vi "WFDC Get Reference Images.vi"(0 "IDS Camera Notifier":string="IDS-Camera-Wide Field Drift Correction-1", 2 "Data Save Path":path=path "C:/Users/George Sirinakis/Documents/Microscope Control/Microscope Modules/Wide Field Drift Correction/WFDC Default Data Storage", 7 "Z Stage Notifier":string="Prior-Stage-Sample Z-Dev1/ao0", 11 "Scan Range":dbl=1.0, 13 "Frame per Step":u32=1, 14 "Scan Positions File Name":string="Scan Positions.xml") -> ()   [LabVIEW 2020]
uses:
  Device Library/Cameras/IDS/IDS Controls/IDS Actions.ctl
  Device Library/Stages/Stages Controls/Stage Actions.ctl
  <vilib>/Utility/miscctls.llb/LVPointTypeDef.ctl
  WFDC Controls/WFDC Reference Image Info.ctl
panel:
  out "Wait Bar":i32(slide) scale=0.0..11.0
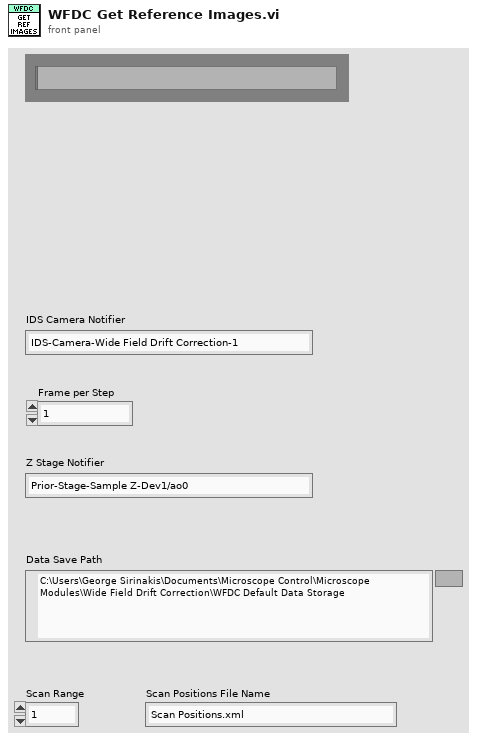
[diagram p1: front panel]
types:
  T1 = typedef "Stage Actions.ctl" = enum16{"Get Position", "MVR", "MOVE", "HALT", "ONTARGET", "ERROR", "REFERENCE", "INIT", "VELOCITY", "STATUS", "EXIT", "HOME", "ZEROPOS", "NANOPOS", "ANALOG", "QUIT"}
  T2 = enum16{"Always On", "Always Off", "Off While Running"}
  T3 = typedef "LVPointTypeDef.ctl" = cluster{"Horizontal":i16, "Vertical":i16}
  T4 = typedef "IDS Actions.ctl" = enum16{"Error Check", "Initialize", "Preview", "Record", "Abort", "Record Settings", "Set Parameter", "Get Parameter", "Set ROI", "Get ROI", "Status", "Quit"}
  T5 = typedef "LVRectTypeDef.ctl" = cluster{"Left":i16, "Top":i16, "Right":i16, "Bottom":i16}
  T6 = typedef "LVBoundsTypeDef.ctl" = cluster{"Width":u32, "Height":u32}
  T7 = typedef "WFDC Reference Image Info.ctl" = cluster{"Image Path":path, "Z Position":dbl, "Number of Frames":u32}
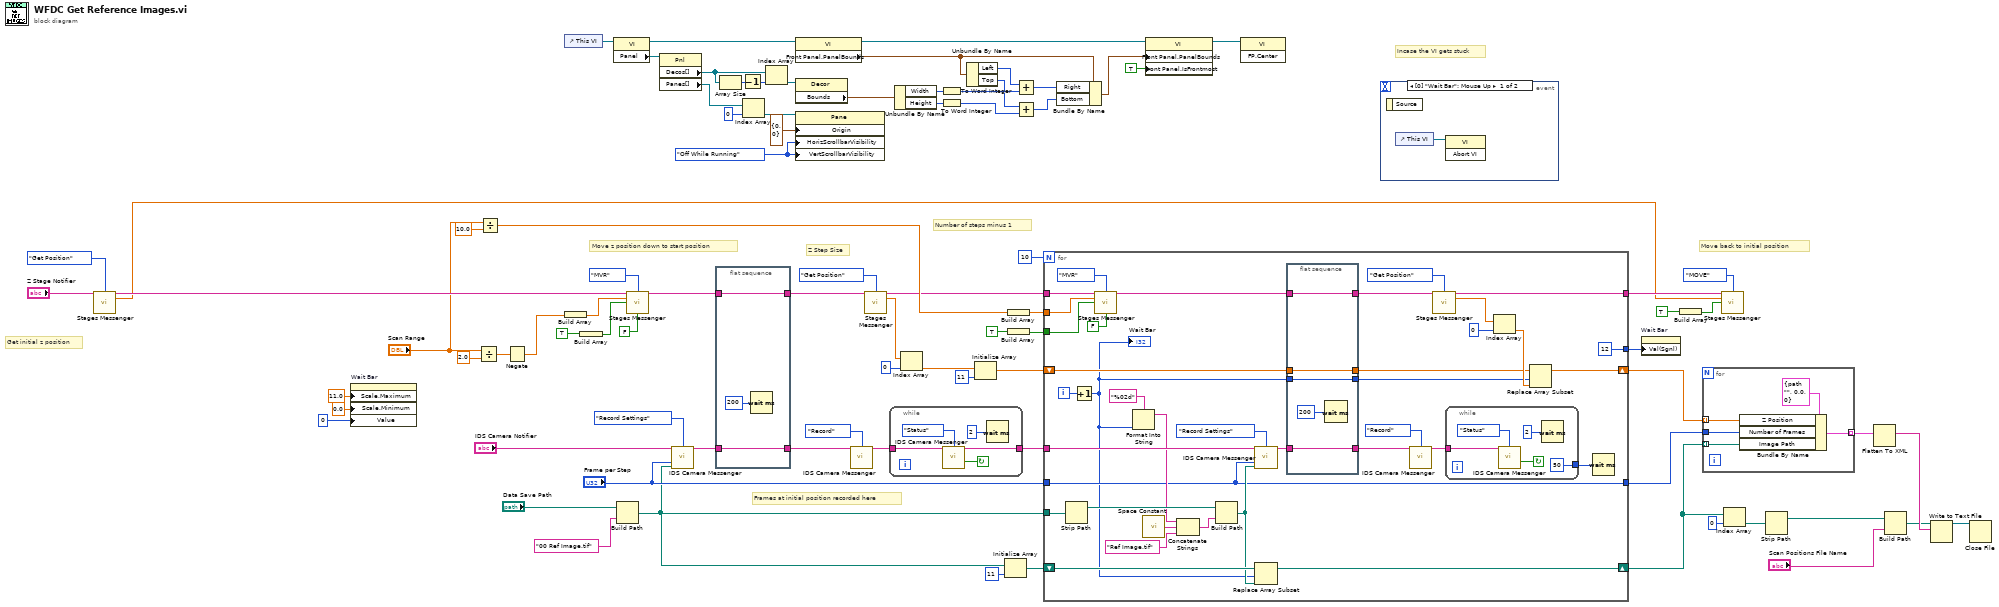
[diagram p0: block diagram]
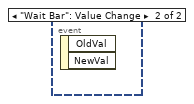
[diagram p2: hidden frame]
diagram:
  w36 = T2."Off While Running" ("Vertical Scrollbar Visibility")
  # "Z Step Size"
  # "Number of steps minus 1"
  # "Frames at initial position recorded here"
  # "Incase the VI gets stuck"
  # "Move back to initial position"
  # "Move z position down to start position"
  # "Get initial z position"
  n1 = call "Stages Messenger.vi"("Stage Notifier Name"="Z Stage Notifier", "Actions"=Stage_Actions."Get Position") -> ("Stage Notifier Name (Dup)"=w77:string, "Positions"=w47:dbl[])  [unwired: 9 in, 3 out]
  n2 = property on="Wait Bar" class="Slide (strict)"("Scale.Maximum"=11.0 ("Scale.Range:Maximum"), "Scale.Minimum"=0.0 ("Scale.Range:Minimum"), "Value"=0 ("Wait Bar")) -> ()  [unwired: 2 in, 2 out]
  n3 = Divide(x="Scan Range", y=2.0) -> (x/y=w13:dbl)
  n4 = Divide(x="Scan Range", y=10.0) -> (x/y=w10:dbl)
  n5 = Negate(x=w13) -> (-x=w14:dbl)
  n6 = control-ref of="This VI"() -> (w19:refnum<vi>)
  n7 = Build Array(w14) -> (w80:dbl[])
  n8 = Build Array(TRUE) -> (w81:bool[])
  n9 = property class="VI"(reference=w19) -> (reference out=w37:refnum<vi>, "Panel"=w30:refnum<vi>)  [unwired: 1 in, 1 out]
  n10 = Build Path(base path="Data Save Path", name or relative path="00 Ref Image.tif") -> (appended path=w59:path)
  n11 = call "Stages Messenger.vi"("Stage Notifier Name"=w77, "Actions"=Stage_Actions."MVR", "Setpoint"=w80, "Axis"=w81, "Exit While Busy?"=FALSE) -> ("Stage Notifier Name (Dup)"=w9:string)  [unwired: 6 in, 4 out]
  n12 = property class="Pnl"(reference=w30) -> ("Decos[]"=w29:refnum<vi>[], "Panes[]"=w33:refnum<vi>[])  [unwired: 1 in, 2 out]
  n13 = call "IDS Camera Messenger.vi"("Notifier Name"="IDS Camera Notifier", "IDS Actions"=IDS_Actions."Record Settings", "# of Frames"="Frame per Step", "File Save Path"=w59) -> ("Notifier Name (Dup)"=w73:string)  [unwired: 6 in, 5 out]
  n14 = flat-sequence {
    tunnel: w9 -> [w89]
    tunnel: [w89] -> w7
    tunnel: w73 -> [w88]
    tunnel: [w88] -> w72
    frame #0 {
      n15 = Wait (ms)(milliseconds to wait=u32 200) -> ()  [unwired: 1 out]
    }
  }
  n16 = Array Size(array=w29) -> (size(s)=w27:i32)
  n17 = Decrement(x=w27) -> (x-1=w28:i32)
  n18 = Index Array(array=w33, index=0) -> (element=w32:refnum<vi>)
  n19 = Index Array(array=w29, index=w28) -> (element=w35:refnum<vi>)
  n20 = property class="VI"(reference=w37) -> (reference out=w39:refnum<vi>, "Front Panel.PanelBounds"=w40:T5)  [unwired: 1 in, 1 out]
  n21 = property class="Decor"(reference=w35) -> ("Bounds"=w38:T6)  [unwired: 1 in, 2 out]
  n22 = property class="Pane"(reference=w32, "Origin"=T3 {"Horizontal"=0, "Vertical"=0}, "HorizScrollbarVisibility"=w36, "VertScrollbarVisibility"=w36) -> ()  [unwired: 1 in, 2 out]
  n23 = call "IDS Camera Messenger.vi"("Notifier Name"=w72, "IDS Actions"=IDS_Actions."Record") -> ("Notifier Name (Dup)"=w49:string)  [unwired: 8 in, 5 out]
  n24 = call "Stages Messenger.vi"("Stage Notifier Name"=w7, "Actions"=Stage_Actions."Get Position") -> ("Stage Notifier Name (Dup)"=w4:string, "Positions"=w6:dbl[])  [unwired: 9 in, 3 out]
  n25 = while {
    tunnel: w49 -> [w93]
    tunnel: [w90] -> w48
    stop <- w92 continue-if-true
    n26 = call "IDS Camera Messenger.vi"("Notifier Name"=w93, "IDS Actions"=IDS_Actions."Status") -> ("Notifier Name (Dup)"=w90:string, "Running?"=w92:bool)  [unwired: 8 in, 4 out]
    n27 = Wait (ms)(milliseconds to wait=u32 2) -> ()  [unwired: 1 out]
  }
  n28 = Unbundle By Name(w38) -> ("Width"=w43:u32, "Height"=w46:u32)
  n29 = Index Array(array=w6, index=0) -> (element=w5:dbl)
  n30 = To Word Integer(number=w43) -> (16bit integer=w45:i16)
  n31 = To Word Integer(number=w46) -> (16bit integer=w24:i16)
  n32 = Unbundle By Name(w40) -> ("Left"=w42:i16, "Top"=w26:i16)
  n33 = Initialize Array(w5, 11 ("dimension size")) -> (w70:dbl[])
  n34 = Initialize Array(w59, 11 ("dimension size")) -> (w58:path[])
  n35 = Build Array(w10) -> (w62:dbl[])
  n36 = Build Array(TRUE) -> (w61:bool[])
  n37 = Add(x=w42, y=w45) -> (x+y=w44:i16)
  n38 = Add(x=w26, y=w24) -> (x+y=w25:i16)
  n39 = for {
    N: 10 -> [_]
    tunnel: w48 -> [w126]
    tunnel: w4 -> [w129]
    shift-right: [w98] -> w57
    shift-left: w70 -> [w104]
    tunnel: w59 -> [w125]
    tunnel: "Frame per Step" -> [w109]
    tunnel: [w97] -> w67
    tunnel: w62 -> [w114]
    tunnel: w61 -> [w113]
    shift-right: [w110] -> w54
    shift-left: w58 -> [w112]
    tunnel: [w109] -> w56
    tunnel: [12 ("Value (Signaling)")] -> w20
    i -> [w128]
    n40 = Strip Path(path=w125) -> (stripped path=w124:path)  [unwired: 1 out]
    n41 = Increment(x=w128) -> (x+1=w96:i32)
    "Wait Bar" <- w96
    n42 = call "Stages Messenger.vi"("Stage Notifier Name"=w129, "Actions"=Stage_Actions."MVR", "Setpoint"=w114, "Axis"=w113, "Exit While Busy?"=FALSE) -> ("Stage Notifier Name (Dup)"=w105:string)  [unwired: 6 in, 4 out]
    n43 = Format Into String(format string="%02d", w96) -> (resulting string=w119:string)  [unwired: 2 in, 1 out]
    n44 = call <vilib>:"Space Constant.vi"() -> ("String"=w123:string)
    n45 = Concatenate Strings(w119, w123, "Ref Image.tif") -> (w121:string)
    n46 = Build Path(base path=w124, name or relative path=w121) -> (appended path=w111:path)
    n47 = call "IDS Camera Messenger.vi"("Notifier Name"=w126, "IDS Actions"=IDS_Actions."Record Settings", "# of Frames"=w109, "File Save Path"=w111) -> ("Notifier Name (Dup)"=w118:string)  [unwired: 6 in, 5 out]
    n48 = Replace Array Subset(array=w112, new element=w111, index=w96) -> (w110:path[])
    n49 = flat-sequence {
      tunnel: w118 -> [w140]
      tunnel: [w141] -> w100
      tunnel: w104 -> [w141]
      tunnel: [w140] -> w117
      tunnel: w105 -> [w138]
      tunnel: [w138] -> w103
      tunnel: w96 -> [w137]
      tunnel: [w137] -> w95
      frame #0 {
        n50 = Wait (ms)(milliseconds to wait=u32 200) -> ()  [unwired: 1 out]
      }
    }
    n51 = call "IDS Camera Messenger.vi"("Notifier Name"=w117, "IDS Actions"=IDS_Actions."Record") -> ("Notifier Name (Dup)"=w115:string)  [unwired: 8 in, 5 out]
    n52 = call "Stages Messenger.vi"("Stage Notifier Name"=w103, "Actions"=Stage_Actions."Get Position") -> ("Stage Notifier Name (Dup)"=w97:string, "Positions"=w99:dbl[])  [unwired: 9 in, 3 out]
    n53 = while {
      tunnel: w115 -> [w135]
      tunnel: [u32 50 ("milliseconds to wait")] -> w108
      stop <- w134 continue-if-true
      n54 = call "IDS Camera Messenger.vi"("Notifier Name"=w135, "IDS Actions"=IDS_Actions."Status") -> ("Running?"=w134:bool)  [unwired: 8 in, 5 out]
      n55 = Wait (ms)(milliseconds to wait=u32 2) -> ()  [unwired: 1 out]
    }
    n56 = Index Array(array=w99, index=0) -> (element=w101:dbl)
    n57 = Replace Array Subset(array=w100, new element=w101, index=w95) -> (w98:dbl[])
    n58 = Wait (ms)(milliseconds to wait=w108) -> ()  [unwired: 1 out]
  }
  n59 = Bundle By Name(cluster=w40, "Right"=w44, "Bottom"=w25) -> (w41:T5)
  n60 = property class="VI"(reference=w39, "Front Panel.PanelBounds"=w41, "Front Panel.IsFrontmost"=TRUE ("Front Panel Window:Is Frontmost")) -> (reference out=w16:refnum<vi>)  [unwired: 1 in, 1 out]
  n61 = invoke class="VI" method="FP.Center"(reference=w16) -> ()  [unwired: 2 in, 3 out]
  n62 = event shown="[0] \"Wait Bar\": Mouse Up" {
    selector: _ -> [_ _]
    dyn-events: _ -> [_ _]
    timeout: _ -> [_ _]
    event "Wait Bar": Mouse Up {
      n63 = event-data() -> ()  [unwired: 1 in, 1 out]
      n64 = control-ref of="This VI"() -> (w142:refnum<vi>)
      n65 = invoke class="VI" method="Abort VI"(reference=w142) -> ()  [unwired: 2 in, 3 out]
    }
    event "Wait Bar": Value Change {
      n66 = event-data() -> ()  [unwired: 1 in, 2 out]
    }
  }
  n67 = property on="Wait Bar" class="Slide (strict)"("Val(Sgnl)"=w20) -> ()  [unwired: 2 in, 2 out]
  n68 = Build Array(TRUE) -> (w64:bool[])
  n69 = for {
    tunnel: w57 -> [w146] mode=indexing
    tunnel: w54 -> [w144] mode=indexing
    tunnel: w56 -> [w145]
    tunnel: [w143] -> w55 mode=indexing
    n70 = Bundle By Name(cluster=T7 {"Image Path"=path "", "Z Position"=0.0, "Number of Frames"=0} ("Reference Image Info"), "Z Position"=w146, "Number of Frames"=w145, "Image Path"=w144) -> (w143:T7)
  }
  n71 = call "Stages Messenger.vi"("Stage Notifier Name"=w67, "Actions"=Stage_Actions."MOVE", "Setpoint"=w47, "Axis"=w64) -> ()  [unwired: 7 in, 5 out]
  n72 = Index Array(array=w54, index=0) -> (element=w52:path)
  n73 = Strip Path(path=w52) -> (stripped path=w3:path)  [unwired: 1 out]
  n74 = Flatten To XML(6:w55) -> (2:w51:string)
  n75 = Build Path(base path=w3, name or relative path="Scan Positions File Name") -> (appended path=w18:path)
  n76 = Write to Text File(file (use dialog)=w18, text=w51) -> (refnum out=w50:refnum<file>)  [unwired: 2 in, 2 out]
  n77 = Close File(refnum=w50) -> ()  [unwired: 1 in, 2 out]
